vi "Algo Tester V3.vi"() -> ()   [LabVIEW 2013]
uses:
  <vilib>/rvi/Emulation/niFpgaSctlEmulationGetInTimedLoop.vi
  <vilib>/rvi/Emulation/niFpgaEmulationReportErrorSimple.vi
  <vilib>/rvi/Emulation/niFpgaGetClockAttributes.vi
  <vilib>/rvi/FIFO/Fifo_Resource/nirvififoEmulationWriteFpgaImpl.vi
  <vilib>/rvi/DataTransferAndStorage/Container/Common/niFpgaContainerGetUniqueNameForEmu.vi
  <vilib>/rvi/Emulation/niFpgaCriticalErrorInLSC.vi
  <vilib>/rvi/Emulation/niFpgaProcessEmulError.vi
  LIDAR V2 Globals.vi
  <vilib>/rvi/DataTransferAndStorage/Container/XNode/niFpgaContainer.xnode
  <vilib>/rvi/FIFO/Fifo_Resource/nirvififoEmulationWrite.vi
panel:
  out "FirstSamp":bool
  in  "Count(Ticks)":u32=3000
  out "MemSelect":bool=TRUE
  out "ForIndex":i32=99
  in  "SampEn":bool=TRUE
  in  "FillMem":bool
  in  "LedIndex":u16=40
  out "LastIterration":bool
  out "FirstIterration":bool
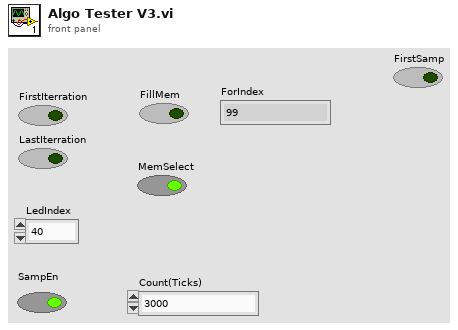
[diagram p1: front panel]
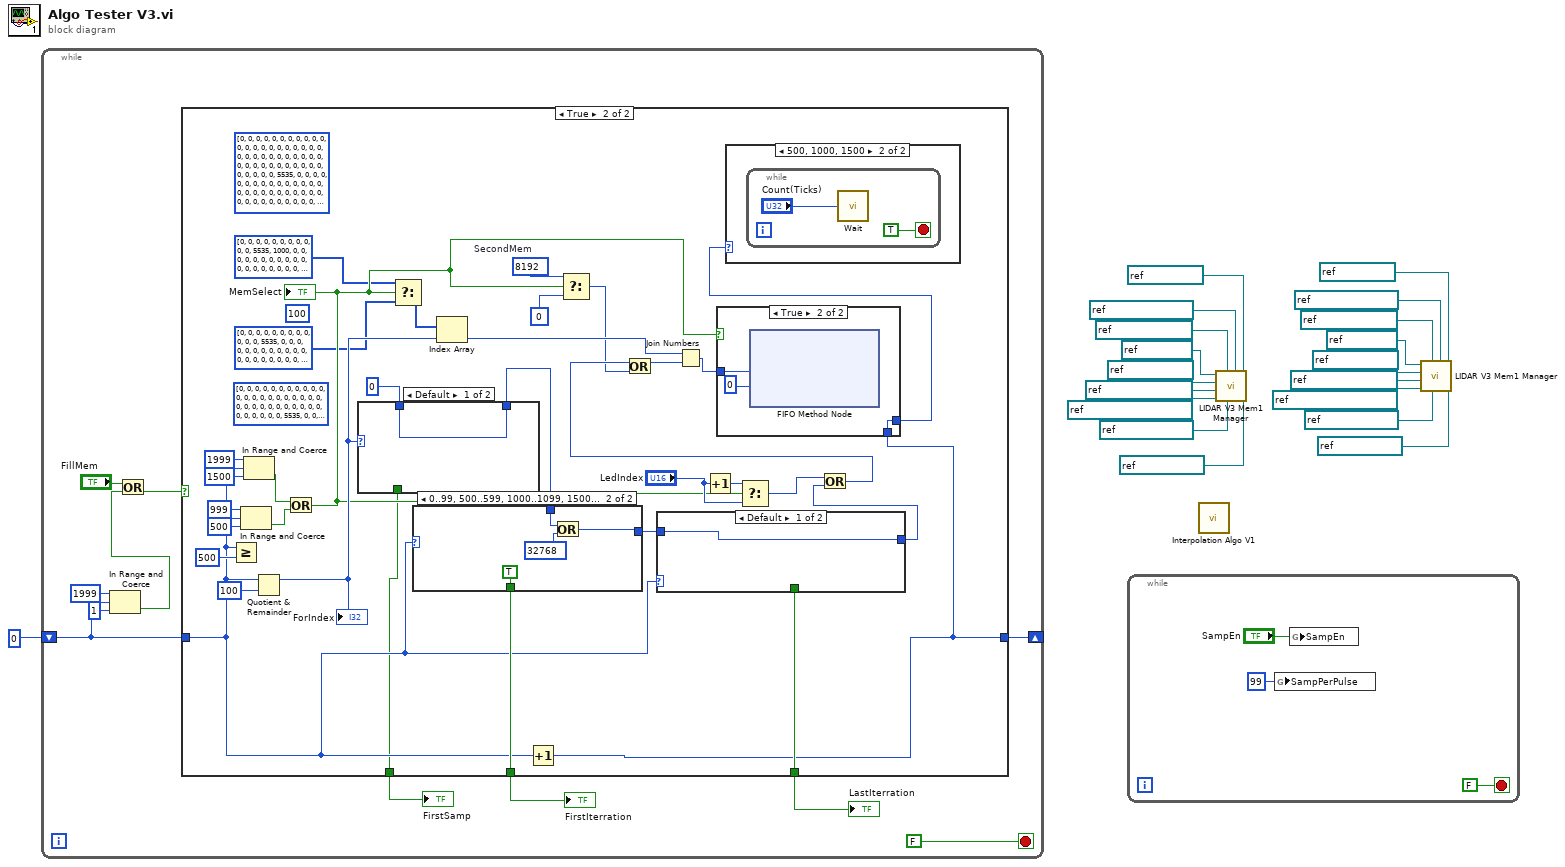
[diagram p0: block diagram]
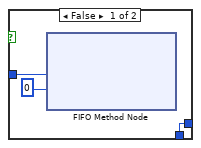
[diagram p4: hidden frame]
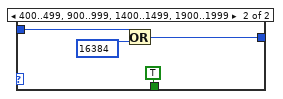
[diagram p5: hidden frame]
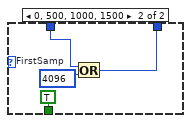
[diagram p7: hidden frame]
diagram:
  n1 = while {
    shift-right: [w27] -> _
    shift-left: i16 0 -> [w26]
    stop <- FALSE stop-if-true
    n2 = In Range and Coerce(upper limit=i16 1999, x=w26, lower limit=i16 1) -> (In Range?=w23:bool)  [unwired: 1 out]
    n3 = Or(x="FillMem", y=w23) -> (x .or. y?=w29:bool)
    n4 = case shown="True" w29 {
      tunnel: w26 -> [_ w36]
      tunnel: [_ w34] -> w27
      tunnel: [_ w38] -> w22
      tunnel: [_ w37] -> w21
      tunnel: [_ w35] -> w20
      frame False {
      }
      frame True {
        (unwired) u16[] [0, 0, 0, 0, 0, 0, 0, 0, 0, 0, 0, 0, 0, 0, 0, 0, 0, 0, 0, 0, 0, 0, 0, 0, 0, 0, 0, 0, 0, 0, 0, 0, 0, 0, 0, 0, 0, 0, 0, 5535, 0, 0, 0, 0, 0, 0, 0, 0, 0, 0, 0, 0, 0, 0, 0, 0, 0, 0, 0, 0, 0, 0, 0, 0, 0, 0, 0, 0, 0, 0, 0, 0, 0, 0, 0, 0, 0, 0, 0, 0, 0, 0, 0, 0, 0, 0, 0, 0, 0, 0, 0, 0, 0, 0, 0, 0, 0, 0, 0, 0]
        (unwired) u16[] [0, 0, 0, 0, 0, 0, 0, 0, 0, 0, 0, 0, 0, 0, 0, 0, 0, 0, 0, 0, 0, 0, 0, 0, 0, 0, 0, 0, 0, 0, 0, 0, 0, 0, 0, 0, 0, 0, 0, 0, 0, 0, 0, 0, 0, 0, 0, 0, 0, 5535, 0, 0, 0, 0, 0, 0, 0, 0, 0, 0, 0, 0, 0, 0, 0, 0, 0, 0, 0, 0, 0, 0, 0, 0, 0, 0, 0, 0, 0, 0, 0, 0, 0, 0, 0, 0, 0, 0, 0, 0, 0, 0, 0, 0, 0, 0, 0, 0, 0, 0]
        w55 = u16 8192  # SecondMem
        (unwired) 100
        n5 = Greater Or Equal?(x=w36, y=i16 500) -> ()  [unwired: 1 out]
        n6 = In Range and Coerce(upper limit=i16 999, x=w36, lower limit=i16 500) -> (In Range?=w41:bool)  [unwired: 1 out]
        n7 = In Range and Coerce(upper limit=i16 1999, x=w36, lower limit=i16 1500) -> (In Range?=w40:bool)  [unwired: 1 out]
        n8 = Quotient & Remainder(x=w36, y=i16 100) -> (x-y*floor(x/y)=w56:i16)  [unwired: 1 out]
        "ForIndex" <- w56
        n9 = Or(x=w40, y=w41) -> (x .or. y?=w39:bool)
        "MemSelect" <- w39
        n10 = case shown="Default" w56 {
          tunnel: u16 0 -> [w82 w85]
          tunnel: [w82 w84] -> w63
          tunnel: [_ TRUE] -> w35
          frame Default {
          }
          frame 0, 500, 1000, 1500 {
            w86 = u16 4096  # FirstSamp
            n11 = Or(x=w85, y=w86) -> (x .or. y?=w84:u16)
          }
        }
        n12 = Select(t=u16[] [0, 0, 0, 0, 0, 0, 0, 0, 0, 0, 0, 5535, 1000, 0, 0, 0, 0, 0, 0, 0, 0, 0, 0, 0, 0, 0, 0, 0, 0, 0, 0, 0, 0, 0, 0, 0, 0, 0, 0, 0, 0, 0, 0, 0, 0, 0, 0, 0, 0, 0, 0, 0, 0, 0, 0, 0, 0, 0, 0, 0, 0, 0, 0, 0, 0, 0, 0, 0, 0, 0, 0, 0, 0, 0, 0, 0, 0, 0, 0, 0, 0, 0, 0, 0, 0, 0, 0, 0, 0, 0, 0, 0, 0, 0, 0, 0, 0, 0, 0, 0], s=w39, f=u16[] [0, 0, 0, 0, 0, 0, 0, 0, 0, 0, 0, 0, 5535, 0, 0, 0, 0, 0, 0, 0, 0, 0, 0, 0, 0, 0, 0, 0, 0, 0, 0, 0, 0, 0, 0, 0, 0, 0, 0, 0, 0, 0, 0, 0, 0, 0, 0, 0, 0, 0, 0, 0, 0, 0, 0, 0, 0, 0, 0, 0, 0, 0, 0, 0, 0, 0, 0, 0, 0, 0, 0, 0, 0, 0, 0, 0, 0, 0, 0, 0, 0, 0, 0, 0, 0, 0, 0, 0, 0, 0, 0, 0, 0, 0, 0, 0, 0, 0, 0, 0]) -> (s? t:f=w51:u16[])
        n13 = case shown="0..99, 500..599, 1000..1099, 1500..1599" w36 {
          tunnel: w63 -> [w77 w80]
          tunnel: [w77 w79] -> w62
          tunnel: [_ TRUE] -> w37
          frame Default {
          }
          frame 0..99, 500..599, 1000..1099, 1500..1599 {
            n14 = Or(x=w80, y=u16 32768) -> (x .or. y?=w79:u16)
          }
        }
        n15 = Index Array(array=w51, index=w56) -> (element=w57:u16)
        n16 = Increment(x=w36) -> (x+1=w34:i16)
        n17 = Select(t=w55, s=w39, f=u16 0 ("SecondMem")) -> (s? t:f=w52:u16)
        n18 = case shown="Default" w36 {
          tunnel: w62 -> [w72 w75]
          tunnel: [w72 w74] -> w61
          tunnel: [_ TRUE] -> w38
          frame Default {
          }
          frame 400..499, 900..999, 1400..1499, 1900..1999 {
            n19 = Or(x=w75, y=u16 16384) -> (x .or. y?=w74:u16)
          }
        }
        n20 = Increment(x="LedIndex") -> (x+1=w46:u16)
        n21 = Select(t=w46, s=w39, f="LedIndex") -> (s? t:f=w48:u16)
        n22 = Or(x=w48, y=w61) -> (x .or. y?=w59:u16)
        n23 = Or(x=w59, y=w52) -> (x .or. y?=w53:u16)
        n24 = Join Numbers(hi=w57, lo=w53) -> ((hi.lo)=w58:u32)
        n25 = case shown="True" w39 {
          tunnel: w58 -> [w68 w70]
          tunnel: [w66 w69] -> w33
          tunnel: w34 -> [w66 w69]
          frame False {
            n26 = xnode ("FIFO Method Node")("Element"=w68, "Timeout"=0) -> ()  [unwired: 1 in, 2 out]
          }
          frame True {
            n27 = xnode ("FIFO Method Node")("Element"=w70, "Timeout"=0) -> ()  [unwired: 1 in, 2 out]
          }
        }
        n28 = case shown="500, 1000, 1500" w33 {
          frame Default {
          }
          frame 500, 1000, 1500 {
            n29 = while {
              stop <- TRUE stop-if-true
              n30 = call "Wait"("Count(Ticks)"="Count(Ticks)") -> ()  [unwired: 1 out]
            }
          }
        }
      }
    }
    "LastIterration" <- w22
    "FirstIterration" <- w21
    "FirstSamp" <- w20
  }
  n31 = while {
    stop <- FALSE stop-if-true
    n32 = global write "LIDAR V2 Globals.vi" "SampPerPulse"(u32 99 ("SampPerPulse")) -> ()
    n33 = global write "LIDAR V2 Globals.vi" "SampEn"("SampEn") -> ()
  }
  n34 = call "Interpolation Algo V1.vi"() -> ()  [unwired: 10 in, 2 out]
  n35 = call "LIDAR V3 Mem1 Manager.vi"("MeanFIFO"=refnum<k21> "MeanVals1", "StartAlgo"=refnum<k21> "StartAlg1", "MemRequest"=refnum<k21> "MemRequest1", "SignalMem"=refnum<k21> "SignalMem1", "MemDataAi"=refnum<k21> "MemDataAi1", "MemRequestDeb"=refnum<k21> "MemRequestDeb1", "MemDataDeb"=refnum<k21> "MemDataDeb1", "MemData"=refnum<k21> "MemData1", "Source Clk"=refnum<k21> "130MHz" ("Source Name")) -> ()  [unwired: 3 in]
  n36 = call "LIDAR V3 Mem1 Manager.vi"("MeanFIFO"=refnum<k21> "MeanVals2", "StartAlgo"=refnum<k21> "StartAlg2", "MemRequest"=refnum<k21> "MemRequest2", "SignalMem"=refnum<k21> "SignalMem2", "MemDataAi"=refnum<k21> "MemDataAi2", "MemRequestDeb"=refnum<k21> "MemRequestDeb2", "MemDataDeb"=refnum<k21> "MemDataDeb2", "MemData"=refnum<k21> "MemData2", "Source Clk"=refnum<k21> "130MHz" ("Source Name")) -> ()  [unwired: 3 in]
